vi "SetODR.vi"(7 "odr":u8, 8 "error in (no error)":errorcluster, 11 "BME680 in":refnum<class "BME680.lvclass">) -> (0 "error out":errorcluster, 3 "BME680 out":refnum<class "BME680.lvclass">)   [LabVIEW 2022 SP3, in "BME680.lvlib" / "BME680.lvclass"]
uses:
  BME680.lvclass
  BME680.lvclass/BME680.ctl
  Typedefs/Conf.ctl
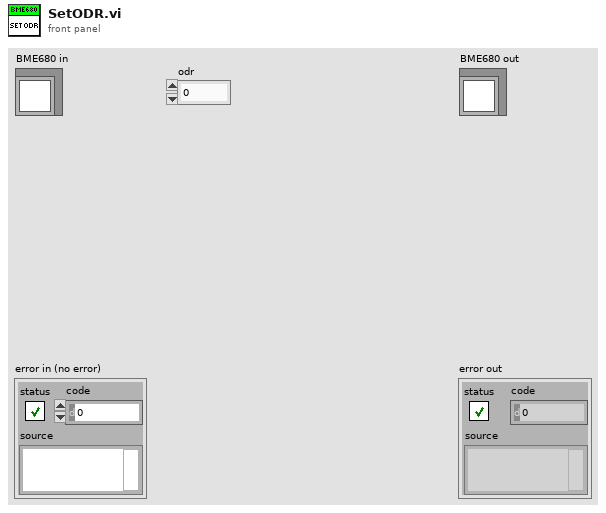
[diagram p1: front panel]
types:
  T1 = typedef "BME680.lvlib/BME680.lvclass/Conf.ctl" = cluster{"os_hum":u8, "os_temp":u8, "os_pres":u8, "filter":u8, "odr":u8}
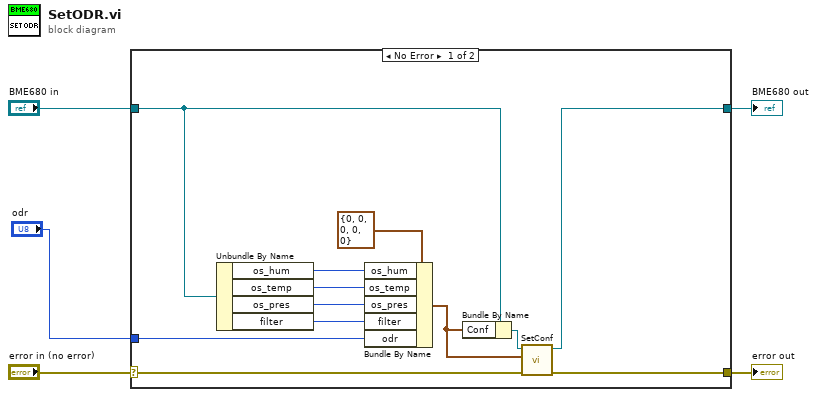
[diagram p0: block diagram]
diagram:
  n1 = case shown="No Error" "error in (no error)" {
    selector: "error in (no error)" -> [w10 w19]
    tunnel: [w9 w19] -> w4
    tunnel: [w7 w18] -> w2
    tunnel: "BME680 in" -> [w8 w18]
    tunnel: "odr" -> [w6 _]
    frame No Error {
      n2 = Unbundle By Name(w8) -> ("os_hum"=w16:u8, "os_temp"=w15:u8, "os_pres"=w14:u8, "filter"=w13:u8)
      n3 = Bundle By Name(cluster=T1 {"os_hum"=0, "os_temp"=0, "os_pres"=0, "filter"=0, "odr"=0} ("Conf"), "os_hum"=w16, "os_temp"=w15, "os_pres"=w14, "filter"=w13, "odr"=w6) -> (w11:T1)
      n4 = Bundle By Name(cluster=w8, "Conf"=w11) -> (w12:refnum<class "BME680.lvclass">)
      n5 = call-dynamic "SetConf.vi"("error in (no error)"=w10, "Conf"=w11, "BME68x in"=w12) -> ("error out"=w9:errorcluster, "BME68x out"=w7:refnum<class "BME680.lvclass">)  [unwired: 7 in]
    }
    frame Error {
    }
  }
  "error out" <- w4
  "BME680 out" <- w2
